vi "Set Shifter (Enum).vi"(8 "error in (no error)":errorcluster, 11 "Shifter":enum16{"Low", "High"}(ring)) -> (0 "error out":errorcluster)   [LabVIEW 2011]
uses:
  Shared/Shifter State.ctl
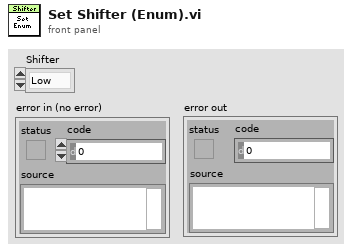
[diagram p1: front panel]
types:
  T1 = typedef "Shifter State.ctl" = enum16{"Unknown", "Low", "High"}
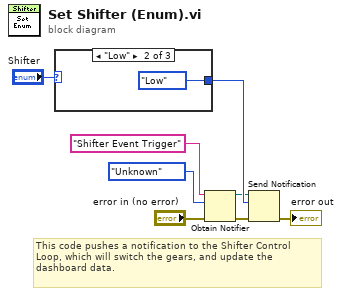
[diagram p0: block diagram]
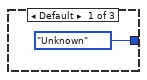
[diagram p2: hidden frame]
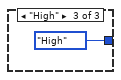
[diagram p3: hidden frame]
diagram:
  # "This code pushes a notification to the Shifter Control Loop, which will switch the gears, and update the dashboard data."
  n1 = case shown="\"Low\"" "Shifter" {
    tunnel: [Shifter_State."Unknown" Shifter_State."Low" Shifter_State."High"] -> w7
    frame Default {
    }
    frame "Low" {
    }
    frame "High" {
    }
  }
  n2 = Obtain Notifier(name (unnamed)="Shifter Event Trigger", notification data type=Shifter_State."Unknown", error in (no error)="error in (no error)") -> (notifier out=w4:refnum<notifier>, error out=w5:errorcluster)  [unwired: 1 in, 1 out]
  n3 = Send Notification(notification=w7, notifier=w4, error in (no error)=w5) -> (error out=→"error out":errorcluster)  [unwired: 1 out]
